vi "Conf COM.vi"(8 "error in (no error)":errorcluster, 11 "Conection Data":T1={"Conection Data"="COM4"}) -> (0 "error out (no error)":errorcluster, 3 "Conection Data 2":T1={"Conection Data"="COM4"})   [LabVIEW 2014, in "AD4212C.lvlib" / "AD4212C.lvclass"]
doc: "Panel de control para configurar el Puerto COM."
uses:
  AD4212CClass/AD4212C.lvclass
  API/Typedef/Connection Data.ctl
  API/AD4212C Lib.lvlib
panel:
  in  "Save Button":bool
  # "Seleccionar Puerto"
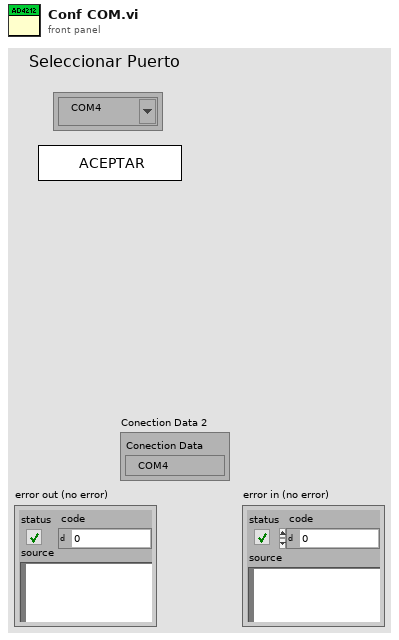
[diagram p1: front panel]
types:
  T1 = typedef "AD4212C Lib.lvlib/Connection Data.ctl" = cluster{"Conection Data":refnum<visa-resource-name>}
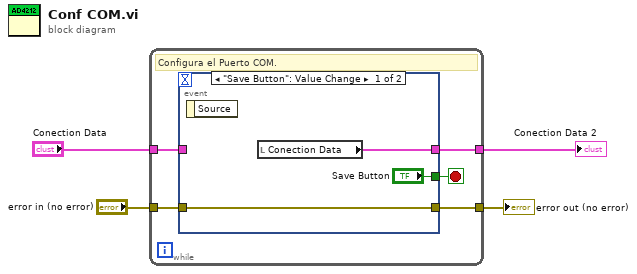
[diagram p0: block diagram]
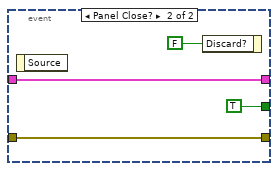
[diagram p2: hidden frame]
diagram:
  n1 = while {
    tunnel: [w8] -> w4
    tunnel: "error in (no error)" -> [w7]
    tunnel: "Conection Data" -> [w6]
    tunnel: [w5] -> w1
    stop <- w9 stop-if-true
    # "Configura el Puerto COM."
    n2 = event shown="[0] \"Save Button\": Value Change" {
      selector: _ -> [_ _]
      dyn-events: _ -> [_ _]
      timeout: _ -> [_ _]
      tunnel: ["Save Button" TRUE ("Save Button")] -> w9
      tunnel: [w11 w14] -> w8
      tunnel: w7 -> [w11 w14]
      tunnel: w6 -> [_ w13]
      tunnel: [w10 w13] -> w5
      event "Save Button": Value Change {
        n3 = event-data() -> ()  [unwired: 1 in, 1 out]
        n4 = local read "Conection Data"() -> (w10:T1)
      }
      event Panel Close? {
        n5 = event-data() -> ()  [unwired: 1 in, 1 out]
        n6 = event-data("Discard?"=FALSE) -> ()  [unwired: 1 in, 1 out]
      }
    }
  }
  "error out (no error)" <- w4
  "Conection Data 2" <- w1
